vi "Delete incoming ObjectInstance Record.vi"(10 "objectInstanceHandle":u64, 11 "Array in":T1[](array[typedef])) -> (2 "Boolean":bool, 3 "Array out":T1[](array[typedef]))   [LabVIEW 2019, in "HLA Custom Device Engine.lvlib"]
uses:
  _typedefs/discoverObjectInstance_type.ctl
  HLA Custom Device Engine.lvlib
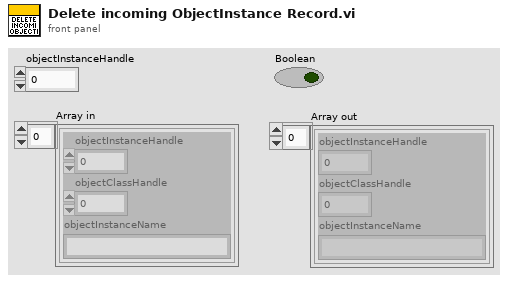
[diagram p1: front panel]
types:
  T1 = typedef "HLA Custom Device Engine.lvlib/discoverObjectInstance_type.ctl" = cluster{"objectInstanceHandle":u64, "objectClassHandle":u64, "objectInstanceName":string}
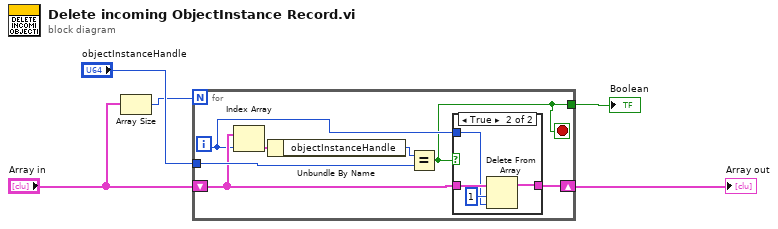
[diagram p0: block diagram]
diagram:
  n1 = Array Size(array="Array in") -> (size(s)=w1:i32)
  n2 = for {
    N: w1 -> [_]
    tunnel: "objectInstanceHandle" -> [w11]
    shift-right: [w7] -> w4
    shift-left: "Array in" -> [w9]
    tunnel: [w6] -> w5
    i -> [w8]
    stop <- w6 stop-if-true
    n3 = Index Array(array=w9, index=w8) -> (element=w10:T1)
    n4 = Unbundle By Name(w10) -> ("objectInstanceHandle"=w12:u64)
    n5 = Equal?(x=w12, y=w11) -> (x = y?=w6:bool)
    n6 = case shown="True" w6 {
      tunnel: w9 -> [w13 w17]
      tunnel: w8 -> [_ w15]
      tunnel: [w13 w14] -> w7
      frame False {
      }
      frame True {
        n7 = Delete From Array(array=w17, length=1, index=w15) -> (array with subset deleted=w14:T1[])  [unwired: 1 out]
      }
    }
  }
  "Boolean" <- w5
  "Array out" <- w4
